vi "OxITC503 _Utility_ Check Instrument Version.vi"(0 "VISA session":refnum<visa-resource-name>, 1 "error in":errorcluster) -> (2 "VISA session out":refnum<visa-resource-name>, 3 "Right Version?":bool, 4 "error out":errorcluster)   [LabVIEW 2013]
doc: "Gets the version string from the instrument and searches in it using the specifier in Version Check."
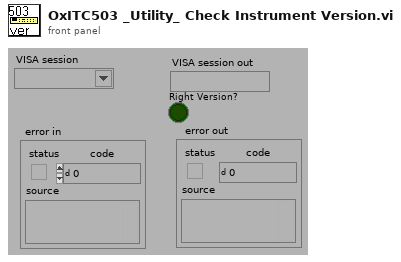
[diagram p1: front panel]
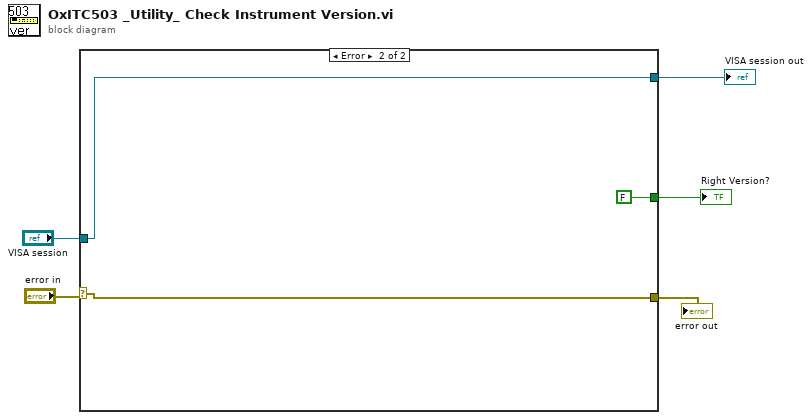
[diagram p0: block diagram]
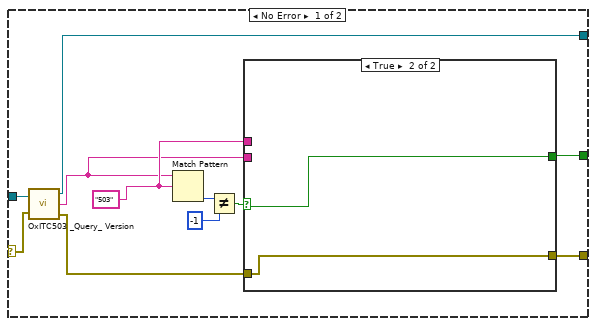
[diagram p2: hidden frame]
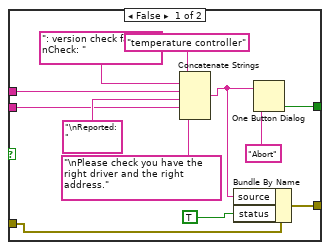
[diagram p3: hidden frame]
diagram:
  n1 = case shown="Error" "error in" {
    selector: "error in" -> [w7 w33]
    tunnel: "VISA session" -> [w13 w32]
    tunnel: [w10 FALSE ("true")] -> w4
    tunnel: [w8 w33] -> w3
    tunnel: [w6 w32] -> w1
    frame No Error {
      w12 = "503" ("regular expression")
      n2 = call "OxITC503 _Query_ Version.vi"("VISA session"=w13, "error in"=w7) -> ("VISA session"=w6:refnum<visa-resource-name>, "Version String"=w11:string, "error out (no error)"=w9:errorcluster)
      n3 = Match Pattern(string=w11, regular expression=w12) -> (offset past match=w16:i32)  [unwired: 1 in, 3 out]
      n4 = Not Equal?(x=w16, y=-1) -> (x != y?=w14:bool)
      n5 = case shown="True" w14 {
        selector: w14 -> [_ w30]
        tunnel: [w22 w30] -> w10
        tunnel: w12 -> [w27 _]
        tunnel: w11 -> [w25 _]
        tunnel: w9 -> [w20 w29]
        tunnel: [w17 w29] -> w8
        frame False {
          n6 = Concatenate Strings("temperature controller", ": version check failure.\nCheck: ", w27, "\nReported: ", w25, "\nPlease check you have the right driver and the right address.") -> (w18:string)
          n7 = Bundle By Name(cluster=w20, "source"=w18, "status"=TRUE) -> (w17:errorcluster)
          n8 = One Button Dialog(message=w18, button name ("OK")="Abort") -> (true=w22:bool)
        }
        frame True {
        }
      }
    }
    frame Error {
    }
  }
  "Right Version?" <- w4
  "error out" <- w3
  "VISA session out" <- w1
